vi "visionFGV.vi"(8 "Error In":errorcluster, 11 "Function":enum16{"set", "read", "close"}(ring)) -> (0 "error out":errorcluster, 3 "Image Out fgv":T1(plugin-control))   [LabVIEW 2019]
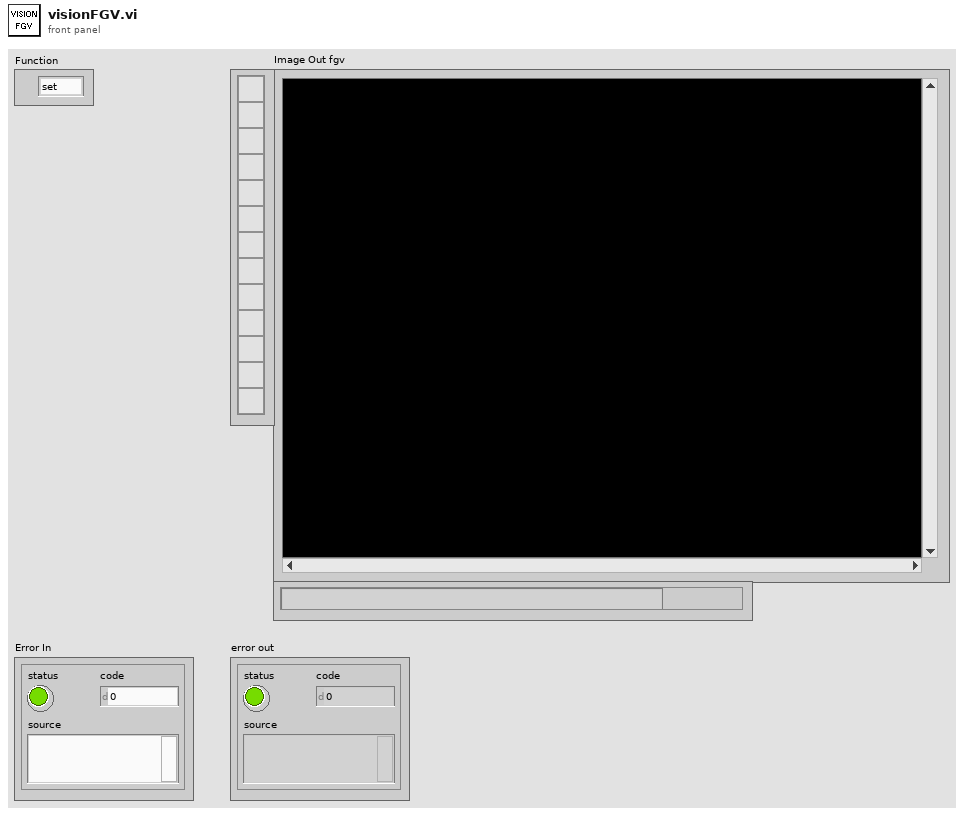
[diagram p1: front panel]
types:
  T1 = typedef "IMAQ Image.ctl" = refnum<image>
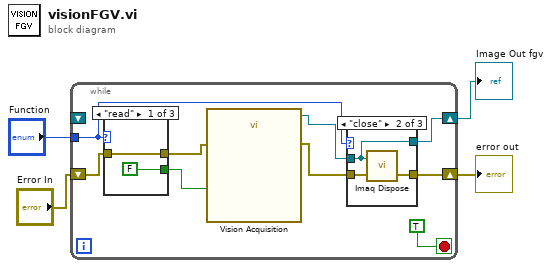
[diagram p0: block diagram]
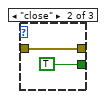
[diagram p4: hidden frame]
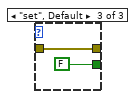
[diagram p5: hidden frame]
diagram:
  n1 = while {
    tunnel: "Function" -> [w9]
    shift-right: [w12] -> w3
    shift-left: "Error In" -> [w11]
    shift-right: [w10] -> w2
    shift-left: _ -> [_]
    stop <- TRUE stop-if-true
    n2 = case shown="\"read\"" w9 {
      tunnel: [w21 w24 w25] -> w8
      tunnel: [FALSE ("Stop (F)") TRUE ("Stop (F)") FALSE ("Stop (F)")] -> w7
      tunnel: w11 -> [w21 w24 w25]
      frame "read" {
      }
      frame "close" {
      }
      frame "set", Default {
      }
    }
    n3 = call "Vision Acquisition"("Stop (F)"=w7, "error in"=w8) -> ("Image Out"=w5:T1, "error out"=w6:errorcluster)  [unwired: 23 in, 1 out]
    n4 = case shown="\"close\"" w9 {
      tunnel: [w15 w18 w19] -> w12
      tunnel: w6 -> [w15 w17 w19]
      tunnel: w5 -> [w14 w16 w20]
      tunnel: [w14 w16 w20] -> w10
      frame "read" {
      }
      frame "close" {
        n5 = call "Imaq Dispose"("Image"=w16, "error in (no error)"=w17) -> ("error out"=w18:errorcluster)  [unwired: 4 in]
      }
      frame Default {
      }
    }
  }
  "Image Out fgv" <- w2
  "error out" <- w3
